vi "GV LL Auth Info.vi"() -> ()   [LabVIEW 2016]
panel:
  in  "Authorization Code":string
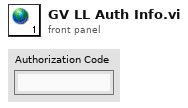
[diagram p1: front panel]
diagram:
